vi "LAB6.vi"() -> ()   [LabVIEW 2011]
uses:
  <userlib>/KNR LabVIEW Toolkit/Type Definitions/Port Number (for US).ctl
  <userlib>/KNR LabVIEW Toolkit/Type Definitions/Port Number (for DC).ctl
  <userlib>/KNR LabVIEW Toolkit/General/KNR Open (Direct Mode).vi
  <vilib>/Utility/inputDevices.llb/closeKeyboard.vi
  <vilib>/Utility/inputDevices.llb/keyboardAcquire.vi
  <userlib>/KNR LabVIEW Toolkit/DC Motor Control/DC Motor Library.lvlib
  <userlib>/KNR LabVIEW Toolkit/Ultrasonic Control/Ultrasonic Library.lvlib
panel:
  out "VR":dbl
  out "VL":dbl
  out "Right (cm)":dbl
  out "Middle(cm)":dbl
  out "Left(cm)":dbl
  out "Ultrasonic output":T1
  in  "Port Number":T2 items=["US1-US4"=0, "US5-US8"=2]
  out "element 2":T3(ring)
  out "element":T3(ring)
  in  "Reverse Encoder 2":bool
  in  "Reset Encoder 2":bool
  in  "Reverse Encoder":bool
  in  "Reset Encoder":bool
  in  "Enable Motor":bool
  out "error out":errorcluster
  in  "stop":bool
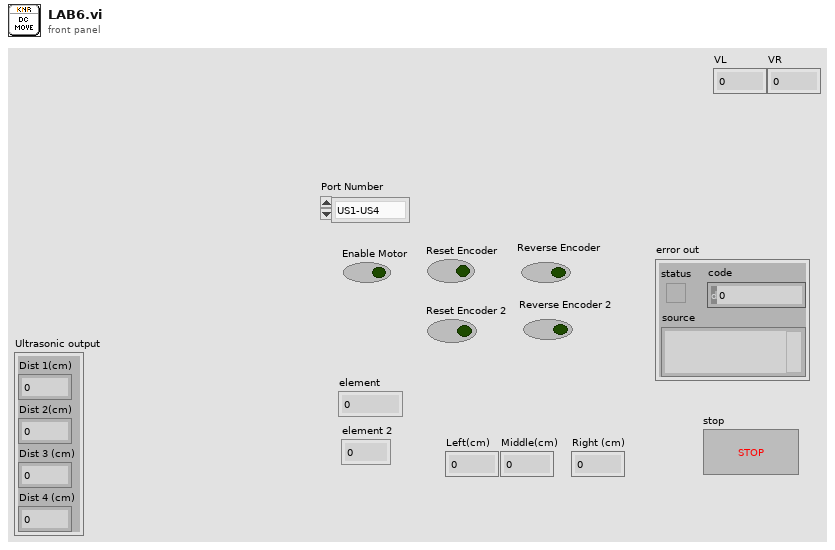
[diagram p1: front panel]
types:
  T1 = cluster{"Dist 1(cm)":dbl, "Dist 2(cm)":dbl, "Dist 3 (cm)":dbl, "Dist 4 (cm)":dbl}
  T2 = typedef "Port Number (for US).ctl" = u16
  T3 = enum16{"0", "1", "2", "3", "4", "5", "6", "7", "8", "9", "A", "B", "C", "D", "E", "F", "G", "H", "I", "J", "K", "L", "M", "N", "O", "P", "Q", "R", "S", "T", "U", "V", "W", "X", "Y", "Z", "F1", "F2", "F3", "F4", "F5", "F6", "F7", "F8", "F9", "F10", "F11", "F12", "F13", "F14", "F15", "ADD", "BACK", "BACKSLASH", "CAPITAL", "COMMA", "DECIMAL", "DELETE", "DIVIDE", "DOWN", "END", "EQUALS", "ESCAPE", "GRAVE (`)", "HOME", "INSERT", "LBRACKET", "LCONTROL", "LEFT", "L ALT", "LSHIFT", "LWIN", "MINUS", "MULTIPLY", "NEXT", "NUMLOCK", "NUMPAD_0", "NUMPAD_1", "NUMPAD_2", "NUMPAD_3", "NUMPAD_4", "NUMPAD_5", "NUMPAD_6", "NUMPAD_7", "NUMPAD_8", "NUMPAD_9", "PAUSE", "PERIOD", "PRIOR (PG UP)", "RBRACKET", "RCONTROL", "RETURN", "RIGHT", "R ALT", "RSHIFT", "RWIN", "SCROLL", "SEMICOLON", "SLASH", "SPACE", "SUBTRACT", "TAB", "UP", "ENTER (num pad)", "' (quote)"}
  T4 = typedef "KNR Reference.ctl" = cluster{"FPGA Session":refnum<class "FPGA Interface Base.lvclass">, "Port Types":T5[]}
  T5 = typedef "Port Type (API).ctl" = enum8{"Unassigned", "DIO", "DC Motor", "RC Motor", "Ultrasonic", "Analog Input"}
  T6 = typedef "Port Number (for DC).ctl" = u16
  T7 = enum16{"0", "1", "2", "3", "4", "5", "6", "7", "8", "9", "A", "B", "C", "D", "E", "F", "G", "H", "I", "J", "K", "L", "M", "N", "O", "P", "Q", "R", "S", "T", "U", "V", "W", "X", "Y", "Z", "F1", "F2", "F3", "F4", "F5", "F6", "F7", "F8", "F9", "F10", "F11", "F12", "F13", "F14", "F15", "ADD", "BACK", "BACKSLASH", "CAPITAL", "COMMA", "DECIMAL", "DELETE", "DIVIDE", "DOWN", "END", "EQUALS", "ESCAPE", "GRAVE (`)", "HOME", "INSERT", "LBRACKET", "LCONTROL", "LEFT", "L ALT", "LSHIFT", "LWIN", "MINUS", "MULTIPLY", "NEXT", "NUMLOCK", "NUMPAD_0", "NUMPAD_1", "NUMPAD_2", "NUMPAD_3", "NUMPAD_4", "NUMPAD_5", "NUMPAD_6", "NUMPAD_7", "NUMPAD_8", "NUMPAD_9", "PAUSE", "PERIOD", "PRIOR (PG UP)", "RBRACKET", "RCONTROL", "RETURN", "RIGHT", "R ALT", "RSHIFT", "RWIN", "SCROLL", "SEMICOLON", "SLASH", "SPACE", "SUBTRACT", "TAB", "UP", "ENTER (num pad)", "' (quote)"}[]
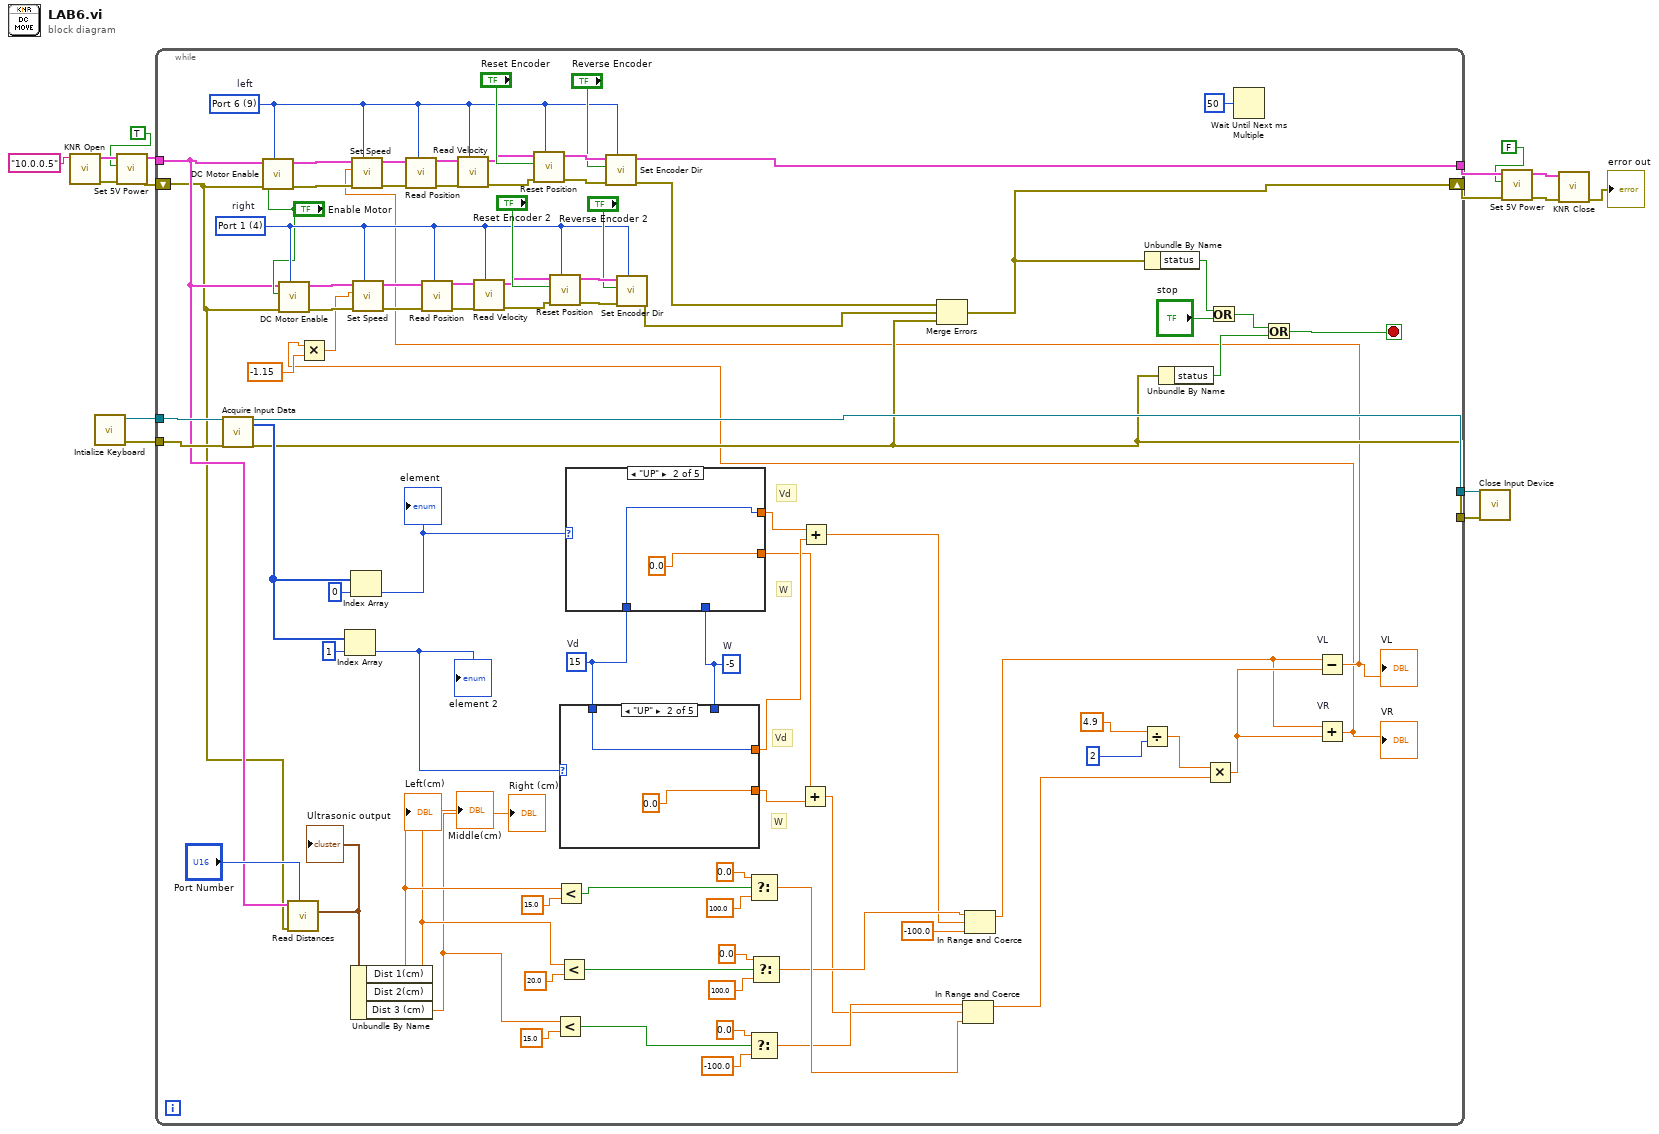
[diagram p0: block diagram]
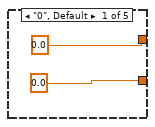
[diagram p2: hidden frame]
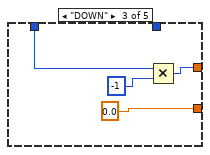
[diagram p3: hidden frame]
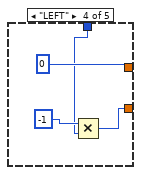
[diagram p4: hidden frame]
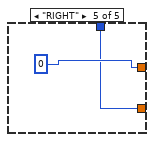
[diagram p5: hidden frame]
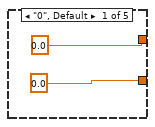
[diagram p6: hidden frame]
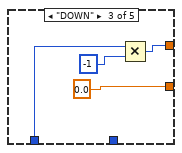
[diagram p7: hidden frame]
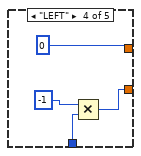
[diagram p8: hidden frame]
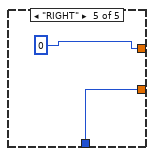
[diagram p9: hidden frame]
diagram:
  n1 = call-poly <userlib>:"KNR Open.vi"("IP Address (Default: 10.0.0.5)"="10.0.0.5") -> ("error out"=w15:errorcluster, "KNR Out"=w16:T4)  [unwired: 9 in]
  n2 = call <vilib>:"Intialize Keyboard.vi"() -> ("error out"=w3:errorcluster, "device ID"=w4:refnum<k1>)  [unwired: 10 in]
  n3 = call <userlib>:"Set 5V Power.vi"("error in (no error)"=w15, "5V Power"=TRUE, "KNR In"=w16) -> ("error out"=w13:errorcluster, "KNR Out"=w14:T4)  [unwired: 7 in]
  n4 = while {
    tunnel: w14 -> [w51]
    shift-right: [w70] -> w8
    shift-left: w13 -> [w50]
    tunnel: [w75] -> w7
    tunnel: w4 -> [w67]
    tunnel: w3 -> [w66]
    tunnel: [w65] -> w2
    tunnel: [w60] -> w1
    stop <- w68 stop-if-true
    w58 = -5  # W
    w57 = 15  # Vd
    w83 = T6 4 items=["Port 1"=4, "Port 2"=5, "Port 3"=6, "Port 4"=7, "Port 5"=8, "Port 6"=9, "Port 7"=10]  # right
    w96 = T6 9 items=["Port 1"=4, "Port 2"=5, "Port 3"=6, "Port 4"=7, "Port 5"=8, "Port 6"=9, "Port 7"=10]  # left
    # "W"
    # "Vd"
    # "W"
    # "Vd"
    n5 = call-poly <vilib>:"Acquire Input Data.vi"("device ID"=w67, "error in (no error)"=w66) -> ("device ID"=w65:refnum<k1>, "keys pressed"=w63:T7, "error out"=w60:errorcluster)  [unwired: 15 in]
    n6 = call <userlib>:"DC Motor Enable.vi"("Port Number"=w96, "error in (no error)"=w50, "Enable Motor"="Enable Motor", "KNR In"=w51) -> ("error out"=w97:errorcluster, "KNR Out"=w98:T4)  [unwired: 6 in]
    n7 = call <userlib>:"DC Motor Enable.vi"("Port Number"=w83, "error in (no error)"=w50, "Enable Motor"="Enable Motor", "KNR In"=w51) -> ("error out"=w84:errorcluster, "KNR Out"=w85:T4)  [unwired: 6 in]
    n8 = call <userlib>:"Read Distances.vi"("Port Number"="Port Number", "error in (no error)"=w50, "KNR In"=w51) -> ("Ultrasonic output"=w52:T1)  [unwired: 6 in, 2 out]
    "Ultrasonic output" <- w52
    n9 = Index Array(array=w63, index=1) -> (element=w56:T3)
    "element 2" <- w56
    n10 = Index Array(array=w63, index=0) -> (element=w59:T3)
    "element" <- w59
    n11 = Unbundle By Name(w52) -> ("Dist 1(cm)"=w46:dbl, "Dist 2(cm)"=w45:dbl, "Dist 3 (cm)"=w44:dbl)
    "Left(cm)" <- w46
    "Middle(cm)" <- w45
    "Right (cm)" <- w44
    n12 = Less?(x=w44, y=15.0) -> (x < y?=w35:bool)
    n13 = Less?(x=w46, y=15.0) -> (x < y?=w37:bool)
    n14 = Less?(x=w45, y=20.0) -> (x < y?=w36:bool)
    n15 = case shown="\"UP\"" w56 {
      tunnel: [0.0 ("Vd") w106 w109 0 0] -> w25
      tunnel: [0.0 ("W") 0.0 ("W") 0.0 ("W") w113 w116] -> w23
      tunnel: w58 -> [_ _ _ w112 w116]
      tunnel: w57 -> [_ w106 w108 _ _]
      frame "0", Default {
      }
      frame "UP" {
      }
      frame "DOWN" {
        n16 = Multiply(x=w108, y=-1 ("W")) -> (x*y=w109:i32)
      }
      frame "LEFT" {
        n17 = Multiply(x=-1, y=w112) -> (x*y=w113:i32)
      }
      frame "RIGHT" {
      }
    }
    n18 = case shown="\"UP\"" w59 {
      tunnel: [0.0 ("Vd") w120 w122 0 0] -> w26
      tunnel: [0.0 ("W") 0.0 ("W") 0.0 ("W") w126 w130] -> w24
      tunnel: w57 -> [_ w120 w124 _ _]
      tunnel: w58 -> [_ _ _ w127 w130]
      frame "0", Default {
      }
      frame "UP" {
      }
      frame "DOWN" {
        n19 = Multiply(x=w124, y=-1 ("W")) -> (x*y=w122:i32)
      }
      frame "LEFT" {
        n20 = Multiply(x=-1, y=w127) -> (x*y=w126:i32)
      }
      frame "RIGHT" {
      }
    }
    n21 = Select(t=0.0 ("y"), s=w37, f=100.0 ("y")) -> (s? t:f=w34:dbl)
    n22 = Select(t=0.0 ("y"), s=w35, f=-100.0 ("y")) -> (s? t:f=w33:dbl)
    n23 = Select(t=0.0 ("y"), s=w36, f=100.0 ("y")) -> (s? t:f=w32:dbl)
    n24 = Add(x=w24, y=w23) -> (x+y=w21:dbl)
    n25 = Add(x=w26, y=w25) -> (x+y=w22:dbl)
    n26 = In Range and Coerce(upper limit=w33, x=w21, lower limit=w34) -> (coerced(x)=w20:dbl)  [unwired: 1 out]
    n27 = In Range and Coerce(upper limit=w32, x=w22, lower limit=-100.0 ("y")) -> (coerced(x)=w19:dbl)  [unwired: 1 out]
    n28 = Divide(x=4.9 ("Vd"), y=2 ("Vd")) -> (x/y=w28:dbl)
    n29 = Unbundle By Name(w60) -> ("status"=w64:bool)
    n30 = Multiply(x=w28, y=w20) -> (x*y=w27:dbl)
    n31 = Wait Until Next ms Multiple(millisecond multiple=u32 50) -> ()  [unwired: 1 out]
    n32 = Subtract "VL"(x=w19, y=w27) -> (x-y=w18:dbl)
    "VL" <- w18
    n33 = call <userlib>:"Set Speed.vi"("Port Number"=w96, "error in (no error)"=w97, "Speed (+-100%)"=w18, "KNR In"=w98) -> ("error out"=w94:errorcluster, "KNR Out"=w95:T4)  [unwired: 6 in]
    n34 = call <userlib>:"Read Position.vi"("Port Number"=w96, "error in (no error)"=w94, "KNR In"=w95) -> ("error out"=w92:errorcluster, "KNR Out"=w93:T4)  [unwired: 6 in, 1 out]
    n35 = call <userlib>:"Read Velocity.vi"("Port Number"=w96, "error in (no error)"=w92, "KNR In"=w93) -> ("error out"=w90:errorcluster, "KNR Out"=w91:T4)  [unwired: 6 in, 1 out]
    n36 = call <userlib>:"Reset Position.vi"("Port Number"=w96, "error in (no error)"=w90, "Reset"="Reset Encoder", "KNR In"=w91) -> ("error out"=w101:errorcluster, "KNR Out"=w102:T4)  [unwired: 6 in]
    n37 = call <userlib>:"Set Encoder Dir.vi"("Port Number"=w96, "error in (no error)"=w101, "Reverse?"="Reverse Encoder", "KNR In"=w102) -> ("error out"=w74:errorcluster, "KNR Out"=w75:T4)  [unwired: 6 in]
    n38 = Add "VR"(x=w19, y=w27) -> (x+y=w17:dbl)
    "VR" <- w17
    n39 = Multiply(x=w17, y=-1.15) -> (x*y=w54:dbl)
    n40 = call <userlib>:"Set Speed.vi"("Port Number"=w83, "error in (no error)"=w84, "Speed (+-100%)"=w54, "KNR In"=w85) -> ("error out"=w81:errorcluster, "KNR Out"=w82:T4)  [unwired: 6 in]
    n41 = call <userlib>:"Read Position.vi"("Port Number"=w83, "error in (no error)"=w81, "KNR In"=w82) -> ("error out"=w79:errorcluster, "KNR Out"=w80:T4)  [unwired: 6 in, 1 out]
    n42 = call <userlib>:"Read Velocity.vi"("Port Number"=w83, "error in (no error)"=w79, "KNR In"=w80) -> ("error out"=w77:errorcluster, "KNR Out"=w78:T4)  [unwired: 6 in, 1 out]
    n43 = call <userlib>:"Reset Position.vi"("Port Number"=w83, "error in (no error)"=w77, "Reset"="Reset Encoder 2", "KNR In"=w78) -> ("error out"=w88:errorcluster, "KNR Out"=w89:T4)  [unwired: 6 in]
    n44 = call <userlib>:"Set Encoder Dir.vi"("Port Number"=w83, "error in (no error)"=w88, "Reverse?"="Reverse Encoder 2", "KNR In"=w89) -> ("error out"=w73:errorcluster)  [unwired: 6 in, 1 out]
    n45 = Merge Errors(w74, w73, w60) -> (w70:errorcluster)
    n46 = Unbundle By Name(w70) -> ("status"=w71:bool)
    n47 = Or(x=w71, y="stop") -> (x .or. y?=w69:bool)
    n48 = Or(x=w69, y=w64) -> (x .or. y?=w68:bool)
  }
  n49 = call-poly <vilib>:"Close Input Device.vi"("error in (no error)"=w1, "device ID"=w2) -> ()  [unwired: 8 in, 1 out]
  n50 = call <userlib>:"Set 5V Power.vi"("error in (no error)"=w8, "5V Power"=FALSE, "KNR In"=w7) -> ("error out"=w10:errorcluster, "KNR Out"=w11:T4)  [unwired: 7 in]
  n51 = call <userlib>:"KNR Close.vi"("error in (no error)"=w10, "KNR In"=w11) -> ("error out"=→"error out":errorcluster)  [unwired: 9 in]
